vi "DL-Read Data Log.vi"(0 "Header in":T1, 7 "First":i32, 9 "N":i32=1, 11 "error in (no error)":errorcluster) -> (4 "Header out":T1, 8 "Array":dbl[][](array[numeric]), 15 "error out":errorcluster)   [LabVIEW 2015]
uses:
  Typedefs/DL-File Header.ctl
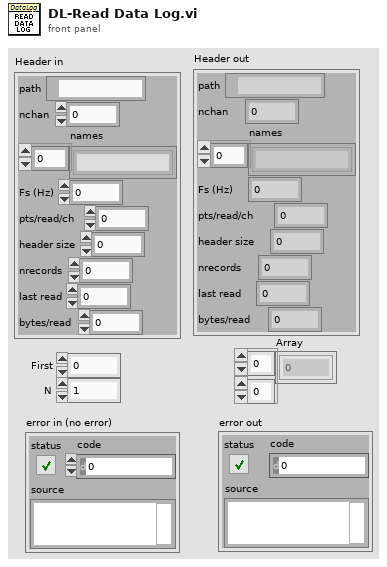
[diagram p1: front panel]
types:
  T1 = typedef "DL-File Header.ctl" = cluster{"path":path, "nchan":i32, "names":string[], "Fs (Hz)":dbl, "pts/read/ch":i32, "header size":i32, "nrecords":i32, "last read":i32, "bytes/read":i32}
  T2 = enum16{"open", "replace", "create", "open or create", "replace or create", "replace or create with confirmation"}
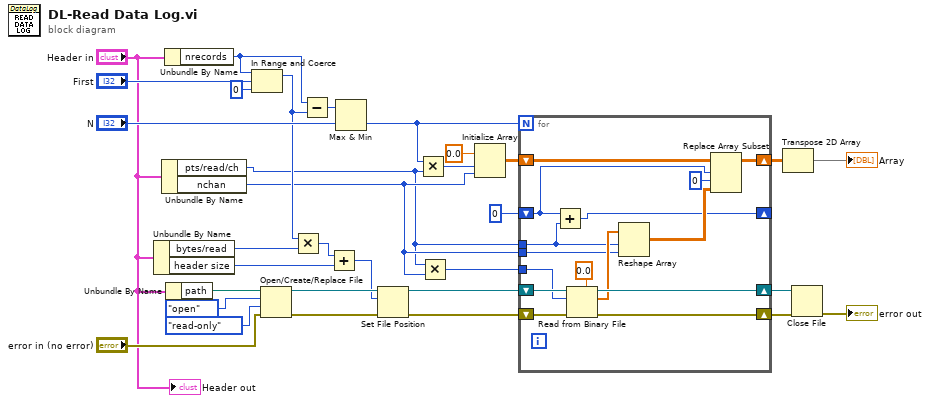
[diagram p0: block diagram]
diagram:
  n1 = Unbundle By Name("Header in") -> ("bytes/read"=w15:i32, "header size"=w13:i32)
  n2 = Unbundle By Name("Header in") -> ("pts/read/ch"=w4:i32, "nchan"=w5:i32)
  n3 = Unbundle By Name("Header in") -> ("nrecords"=w26:i32)
  n4 = Unbundle By Name("Header in") -> ("path"=w30:path)
  n5 = In Range and Coerce(upper limit=w26, x="First", lower limit=0) -> (coerced(x)=w16:i32)  [unwired: 1 out]
  n6 = Open/Create/Replace File(file path (use dialog)=w30, error in="error in (no error)", operation (0:open)=T2."open", access (0:read/write)=enum16{"read/write", "read-only", "write-only"}."read-only") -> (refnum out=w21:refnum<file>, error out=w20:errorcluster)  [unwired: 2 in, 1 out]
  n7 = Multiply(x=w16, y=w15) -> (x*y=w14:i32)
  n8 = Subtract(x=w26, y=w16) -> (x-y=w25:i32)
  n9 = Add(x=w14, y=w13) -> (x+y=w12:i32)
  n10 = Max & Min(x=w25, y="N") -> (min(x,y)=w7:i32)  [unwired: 1 out]
  n11 = Set File Position(offset (in bytes) (0)=w12, refnum=w21, error in=w20) -> (refnum out=w22:refnum<file>, error out=w23:errorcluster)  [unwired: 1 in]
  n12 = Multiply(x=w7, y=w4) -> (x*y=w8:i32)
  n13 = Multiply(x=w4, y=w5) -> (x*y=w6:i32)
  n14 = Initialize Array(0.0, w8, w5) -> (w10:dbl[][])
  n15 = for {
    N: w7 -> [_]
    shift-right: [w44] -> w19
    shift-left: w22 -> [w47]
    shift-right: [w43] -> w18
    shift-left: w23 -> [w46]
    shift-right: [w39] -> w2
    shift-left: w10 -> [w38]
    tunnel: w6 -> [w42]
    tunnel: w5 -> [w40]
    tunnel: w4 -> [w34]
    shift-right: [w33] -> _
    shift-left: 0 -> [w35]
    n16 = Add(x=w35, y=w34) -> (x+y=w33:i32)
    n17 = Read from Binary File(5:0.0, 8:w46, 10:w42, 11:w47) -> (0:w43:errorcluster, 2:w41:dbl[], 3:w44:refnum<file>)  [unwired: 2 in, 1 out]
    n18 = Reshape Array(w41, w34, w40) -> (w37:dbl[][])
    n19 = Replace Array Subset(array=w38, new element=w37, index (row)=w35, index (col)=0 ("disabled index (col)")) -> (w39:dbl[][])
  }
  n20 = Transpose 2D Array(2D array=w2) -> (transposed array=→"Array":dbl[][])
  n21 = Close File(refnum=w19, error in=w18) -> (error out=→"error out":errorcluster)  [unwired: 1 out]
  "Header out" <- "Header in"
